vi "MyG#G3Templ_SetModifiedAttributes.vi"(0 "reference in":refnum<class "MyG#G3Templ.lvclass">, 2 "attributes":T1, 3 "Only unlock data? (F)":bool, 4 "Unlock data if error? (T)":bool=TRUE, 5 "error in (no error)":errorcluster, 7 "Update data even if error? (F)":bool) -> (14 "reference out":refnum<class "MyG#G3Templ.lvclass">, 19 "error out":errorcluster)   [LabVIEW 2020, in "MyG#G3Templ.lvclass"]
doc: "This VI overwrites the class attributes associated with this class or subclass object reference and unlocks it for write access. If error in is set, the object is unlocked but its data will not be modified. If reference is wired, the class attributes of the class (or sub class) will be affected else the class attributes will default to the class.\n\nIn order to use this VI, you must first successfully lock the object's data using this class GetClassAttributesToModify VI."
uses:
  MyG#G3Templ.lvclass
  protected/ObjectAttributes.ctl
  ObjectAttributesRef.ctl
  MyG#G3Templ.lvclass/MyG#G3Templ.ctl
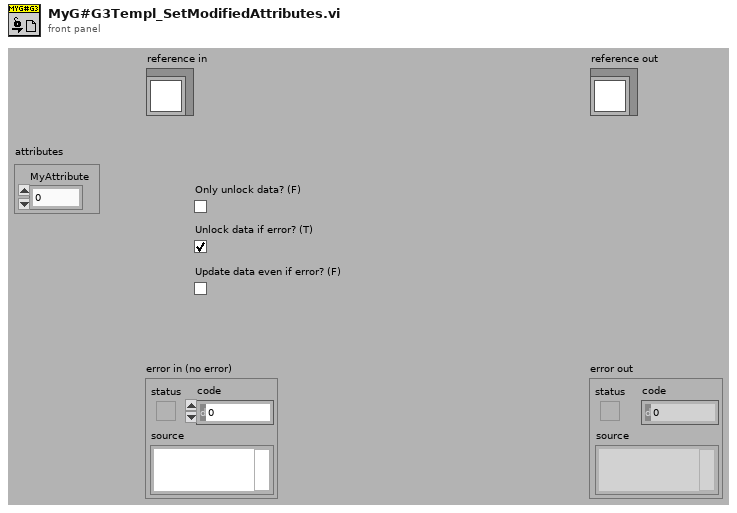
[diagram p1: front panel]
types:
  T1 = typedef "MyG#G3Templ.lvclass/ObjectAttributes.ctl" = cluster{"MyAttribute":dbl}
  T2 = typedef "MyG#G3Templ.lvclass/ObjectAttributesRef.ctl" = refnum<data-value>
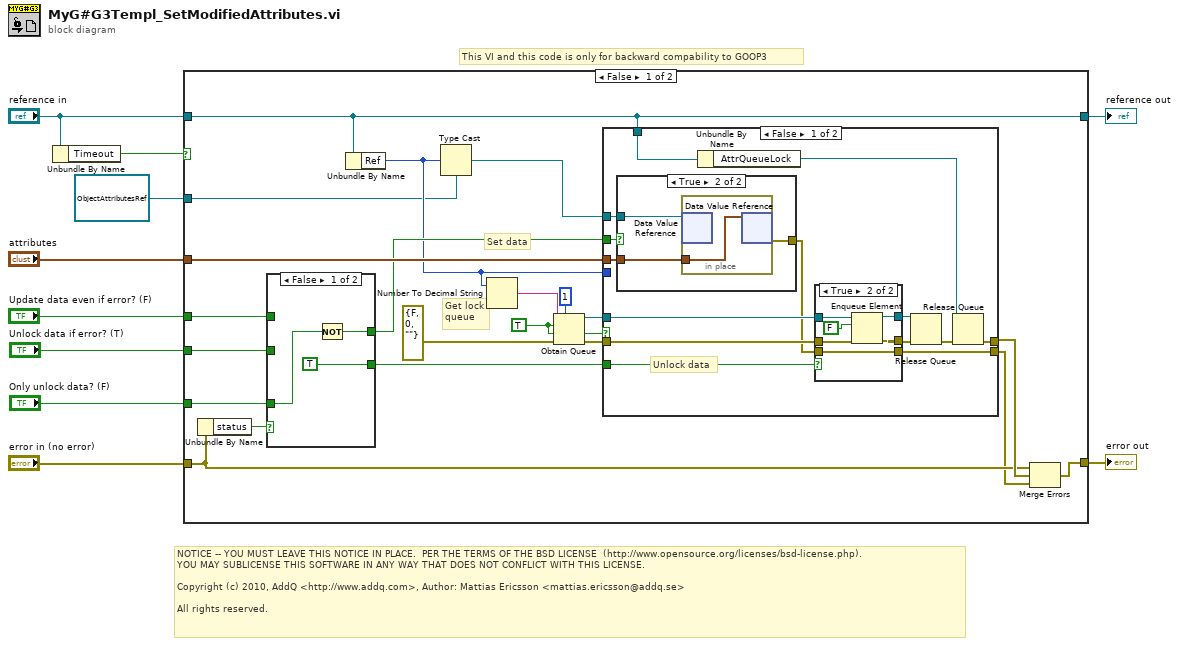
[diagram p0: block diagram]
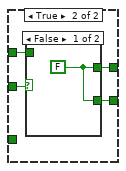
[diagram p2: hidden frame]
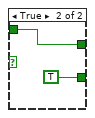
[diagram p3: hidden frame]
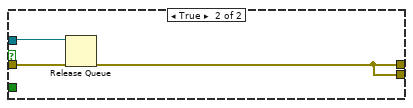
[diagram p6: hidden frame]
diagram:
  # "NOTICE -- YOU MUST LEAVE THIS NOTICE IN PLACE.  PER THE TERMS OF THE BSD LICENSE  (http://www.opensource.org/licenses/bsd-license.php).\nYOU MAY SUBLICENSE THIS SOFTWARE IN ANY WAY THAT DOES NOT CONFLICT WITH THIS LICENSE.\n\nCopyright (c) 2010, AddQ <http://www.addq.com>, Author: Mattias Ericsson <mattias.ericsson@addq.se>\n\nAll rights reserved."
  # "This VI and this code is only for backward compability to GOOP3"
  n1 = Unbundle By Name("reference in") -> ("Timeout"=w2:bool)
  n2 = case shown="False" w2 {
    tunnel: "attributes" -> [w25 _]
    tunnel: [w24 w73] -> w9
    tunnel: "error in (no error)" -> [w23 w73]
    tunnel: "Only unlock data? (F)" -> [w21 _]
    tunnel: "Unlock data if error? (T)" -> [w18 _]
    tunnel: "Update data even if error? (F)" -> [w17 _]
    tunnel: "reference in" -> [w15 w74]
    tunnel: [w15 w74] -> w3
    tunnel: T2 refnum ("attributes ref") -> [w12 _]
    frame False {
      w31 = TRUE ("create if not found? (T)")
      # "Get lock\nqueue"
      # "Set data"
      n3 = Unbundle By Name(w23) -> ("status"=w22:bool)
      n4 = case shown="False" w22 {
        tunnel: [w33 w38] -> w20
        tunnel: w21 -> [w35 _]
        tunnel: [TRUE w37] -> w19
        tunnel: w18 -> [_ w39]
        tunnel: w17 -> [_ w36]
        frame False {
          n5 = Not(x=w35) -> (.not. x?=w33:bool)
        }
        frame True {
          n6 = case shown="False" w39 {
            tunnel: [w40 w41] -> w38
            tunnel: [w40 TRUE] -> w37
            tunnel: w36 -> [_ w41]
            frame False {
              w40 = FALSE
            }
            frame True {
            }
          }
        }
      }
      n7 = Unbundle By Name(w15) -> ("Ref"=w13:u32)
      n8 = Type Cast(type=w12, x=w13) -> (*(type *) &x=w11:T2)
      n9 = Number To Decimal String(number=w13) -> (decimal integer string=w32:string)  [unwired: 1 in]
      n10 = Obtain Queue(max queue size (-1, unlimited)=1, name (unnamed)=w32, element data type=w31, create if not found? (T)=w31, error in (no error)=errorcluster {"status"=FALSE, "code"=0, "source"=""}) -> (queue out=w27:refnum<queue>, created new?=w28:bool, error out=w29:errorcluster)
      n11 = case shown="False" w28 {
        tunnel: w29 -> [w56 w72]
        tunnel: w27 -> [w55 w70]
        tunnel: [w49 w71] -> w26
        tunnel: w13 -> [_ _]
        tunnel: w20 -> [w52 _]
        tunnel: w25 -> [w51 _]
        tunnel: w19 -> [w50 _]
        tunnel: w15 -> [w47 _]
        tunnel: [w44 w71] -> w14
        tunnel: w11 -> [w43 _]
        frame False {
          # "Unlock data"
          n12 = case shown="True" w52 {
            tunnel: w51 -> [_ w68]
            tunnel: [_ w67] -> w45
            tunnel: w43 -> [_ w66]
            frame False {
            }
            frame True {
              n13 = in-place {
                in-place-border: w68 -> [w69]
                n14 = in-place-dvr #1(w66) -> ()  [unwired: 2 out]
                n15 = in-place-dvr #1(w69) -> (w67:errorcluster)  [unwired: 1 out]
              }
            }
          }
          n16 = Unbundle By Name(w47) -> ("AttrQueueLock"=w46:refnum<queue>)
          n17 = case shown="True" w50 {
            tunnel: w56 -> [w58 w65]
            tunnel: w55 -> [w59 w64]
            tunnel: [w58 w63] -> w54
            tunnel: [w59 w62] -> w53
            tunnel: w45 -> [w57 w60]
            tunnel: [w57 w60] -> w44
            frame False {
            }
            frame True {
              n18 = Enqueue Element(queue=w64, element=FALSE, error in (no error)=w65) -> (queue out=w62:refnum<queue>, error out=w63:errorcluster)  [unwired: 1 in, 1 out]
            }
          }
          n19 = Release Queue(queue=w53, error in (no error)=w54) -> (error out=w48:errorcluster)  [unwired: 1 in, 2 out]
          n20 = Release Queue(queue=w46, error in (no error)=w48) -> (error out=w49:errorcluster)  [unwired: 1 in, 2 out]
        }
        frame True {
          n21 = Release Queue(queue=w70, error in (no error)=w72) -> (error out=w71:errorcluster)  [unwired: 1 in, 2 out]
        }
      }
      n22 = Merge Errors(w23, w26, w14) -> (w24:errorcluster)
    }
    frame True {
      # "Timeout!"
    }
  }
  "error out" <- w9
  "reference out" <- w3
